vi "HexapodAcquireHardware.vi"(8 "error in (no error)":errorcluster, 11 "HexapodPI in":refnum<class "HexapodPI.lvclass">) -> (0 "error out":errorcluster, 1 "Status Cluster":T1, 2 "In Motion":bool, 3 "HexapodPI out":refnum<class "HexapodPI.lvclass">, 5 "Array":string[](array[string]))   [LabVIEW 2020, in "HexapodPI.lvclass"]
uses:
  HexapodPI.lvclass
  HexapodPI.lvclass/HexapodPI.ctl
  activeChannel.ctl
  OnOffTypeDef.ctl
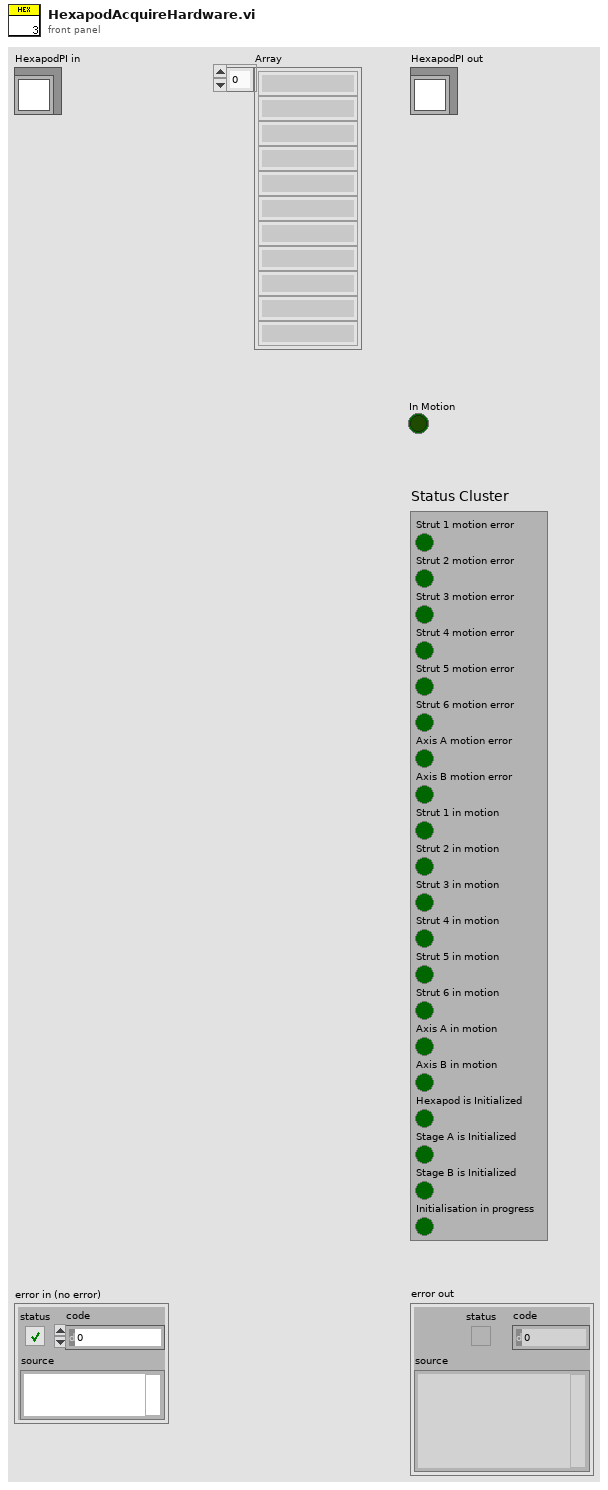
[diagram p1: front panel]
types:
  T1 = cluster{"Strut 1 motion error":bool, "Strut 2 motion error":bool, "Strut 3 motion error":bool, "Strut 4 motion error":bool, "Strut 5 motion error":bool, "Strut 6 motion error":bool, "Axis A motion error":bool, "Axis B motion error":bool, "Strut 1 in motion":bool, "Strut 2 in motion":bool, "Strut 3 in motion":bool, "Strut 4 in motion":bool, "Strut 5 in motion":bool, "Strut 6 in motion":bool, "Axis A in motion":bool, "Axis B in motion":bool, "Hexapod is Initialized":bool, "Stage A is Initialized":bool, "Stage B is Initialized":bool, "Initialisation in progress":bool}
  T2 = enum16{"Not referenced", "Homing", "Moving", "Ready"}
  T3 = typedef "OnOffTypeDef.ctl" = enum16{"off", "on"}
  T4 = cluster{"Zpos":T3, "Zneg":T3, "Xpos":T3, "Xneg":T3, "Ypos":T3, "Yneg":T3, "Wpos":T3, "Wneg":T3, "Vpos":T3, "Vneg":T3, "Upos":T3, "Uneg":T3}
  T5 = cluster{"connection ID":refnum<k5>, "VISA resource name":refnum<visa-resource-name>, "Selector":enum16{"TCPIP", "Serial"}}
  T6 = typedef "activeChannel.ctl" = enum16{"xpos", "ypos", "zpos", "uangle", "vangle", "wangle", "n/a", "off"}
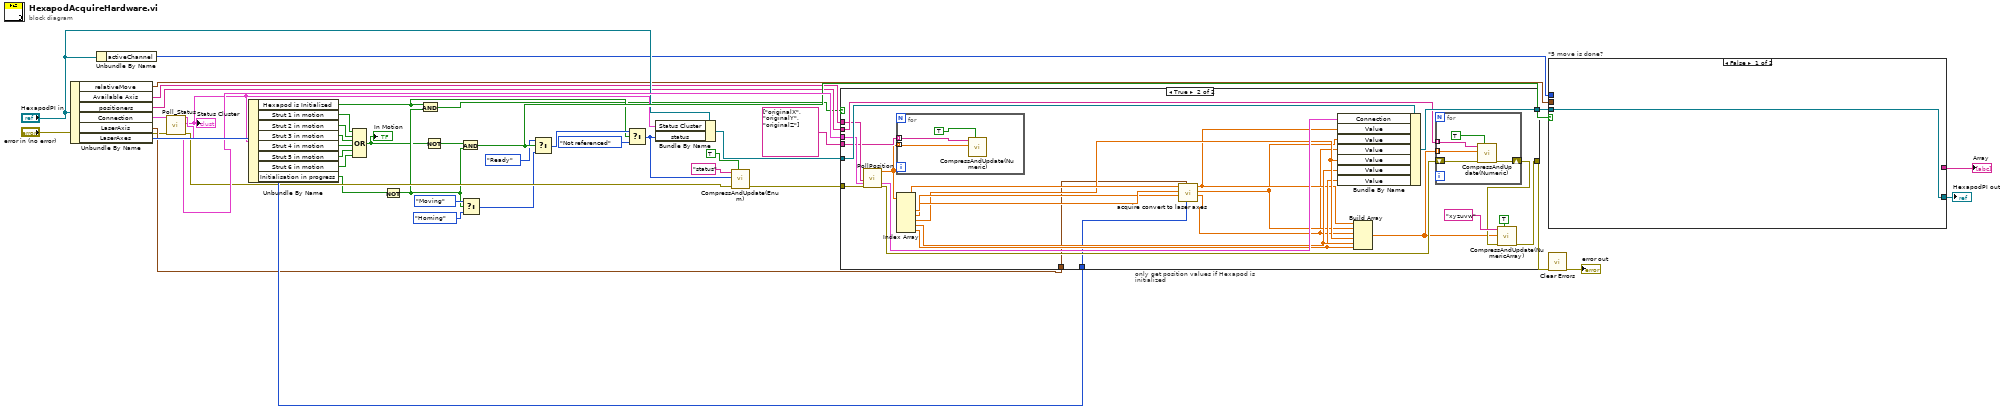
[diagram p0: block diagram]
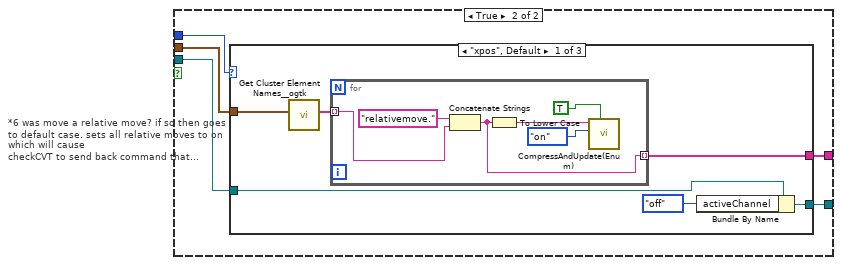
[diagram p2: hidden frame]
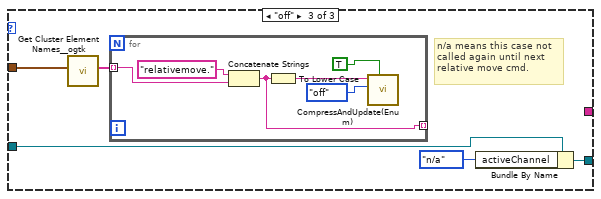
[diagram p4: hidden frame]
diagram:
  n1 = Unbundle By Name("HexapodPI in") -> ("relativeMove"=w33:T4, "Available Axis"=w28:string[], "positioners"=w27:string[], "Connection"=w2:T5, "LaserAxis"=w40:cluster{"u":dbl, "v":dbl, "w":dbl}, "LaserAxes"=w42:T3)
  n2 = Unbundle By Name("HexapodPI in") -> ("activeChannel"=w34:T6)
  n3 = call "Poll_Status.vi"("Connection"=w2, "error in"="error in (no error)") -> ("Connection out"=w41:T5, "Status Cluster"=w29:T1, "error out"=w22:errorcluster)  [unwired: 15 in]
  "Status Cluster" <- w29
  n4 = Unbundle By Name(w29) -> ("Hexapod is Initialized"=w19:bool, "Strut 1 in motion"=w10:bool, "Strut 2 in motion"=w5:bool, "Strut 3 in motion"=w6:bool, "Strut 4 in motion"=w7:bool, "Strut 5 in motion"=w8:bool, "Strut 6 in motion"=w9:bool, "Initialisation in progress"=w4:bool)
  n5 = Compound Arithmetic op=OR(w10, w5, w6, w7, w8, w9) -> (w14:bool)
  "In Motion" <- w14
  n6 = Not(x=w4) -> (.not. x?=w15:bool)
  n7 = And(x=w19, y=w15) -> (x .and. y?=w11:bool)
  n8 = Not(x=w14) -> (.not. x?=w32:bool)
  n9 = And(x=w32, y=w15) -> (x .and. y?=w38:bool)
  n10 = Select(t=T2."Moving" ("Settings.status"), s=w15, f=T2."Homing" ("Settings.status")) -> (s? t:f=w16:T2)
  n11 = Select(t=T2."Ready" ("Settings.status"), s=w38, f=w16) -> (s? t:f=w20:T2)
  n12 = Select(t=w20, s=w19, f=T2."Not referenced" ("Settings.status")) -> (s? t:f=w24:T2)
  n13 = Bundle By Name(cluster="HexapodPI in", "Status Cluster"=w29, "status"=w24) -> (w12:refnum<class "HexapodPI.lvclass">)
  n14 = call "CompressAndUpdate(Enum).vi"("force CVT update (false)"=TRUE, "error in"=w22, "enum variant"=w24, "command or variable name"="status") -> ("error out"=w23:errorcluster)  [unwired: 7 in]
  n15 = case "only get position values if Hexapod is initialized" shown="True" w11 {
    tunnel: [w43 w46] -> w30
    tunnel: [w44 w70] -> w36
    tunnel: w12 -> [w44 w69]
    tunnel: w23 -> [w43 w68]
    tunnel: w41 -> [_ w67]
    tunnel: w27 -> [_ w64]
    tunnel: w28 -> [_ w63]
    tunnel: string[] ["originalX", "originalY", "originalZ"] -> [_ w56]
    tunnel: w40 -> [_ w51]
    tunnel: w42 -> [_ w50]
    frame False {
    }
    frame True {
      n16 = call "PollPosition.vi"("Queried axes"=w63, "Connection"=w67, "error in"=w68) -> ("Position"=w55:dbl[], "Connection out"=w65:T5, "error out"=w66:errorcluster)  [unwired: 13 in, 1 out]
      n17 = for {
        tunnel: w55 -> [w72] mode=indexing
        tunnel: w56 -> [w71] mode=indexing
        n18 = call "CompressAndUpdate(Numeric).vi"("force CVT update (false)"=TRUE, "Numeric"=w72, "command or variable name"=w71) -> ()  [unwired: 8 in, 1 out]
      }
      n19 = Index Array(array=w55) -> (element #1=w62:dbl, element #2=w61:dbl, element #3=w60:dbl, element #4=w59:dbl, element #5=w58:dbl, element #6=w57:dbl)  [unwired: 6 in]
      n20 = call "acquire convert to laser axes.vi"("Settings.Trigger"=w50, "LaserAxis"=w51, "z in"=w60, "y in"=w61, "x in"=w62) -> ("z out"=w52:dbl, "y out"=w53:dbl, "x out"=w54:dbl)  [unwired: 4 in]
      n21 = Bundle By Name(cluster=w69, "Connection"=w65, "Value"=w54, "Value"=w53, "Value"=w52, "Value"=w59, "Value"=w58, "Value"=w57) -> (w70:refnum<class "HexapodPI.lvclass">)
      n22 = Build Array(w54, w53, w52, w59, w58, w57) -> (w45:dbl[])
      n23 = for {
        tunnel: w45 -> [w75] mode=indexing
        tunnel: w64 -> [w74] mode=indexing
        shift-right: [w78] -> w47
        shift-left: w66 -> [w76]
        n24 = call "CompressAndUpdate(Numeric).vi"("force CVT update (false)"=TRUE, "error in"=w76, "Numeric"=w75, "command or variable name"=w74) -> ("error out"=w78:errorcluster)  [unwired: 7 in]
      }
      n25 = call "CompressAndUpdate(NumericArray).vi"("force CVT update (false)"=TRUE, "error in"=w47, "Numeric Array"=w45, "command or variable name"="xyzuvw") -> ("error out"=w46:errorcluster)  [unwired: 7 in]
    }
  }
  n26 = case "*5 move is done?" shown="False" w38 {
    tunnel: w33 -> [_ w84]
    tunnel: w34 -> [_ w83]
    tunnel: w36 -> [w79 w82]
    tunnel: [w79 w81] -> w37
    tunnel: [_ w80] -> w1
    frame False {
    }
    frame True {
      n27 = case "*6 was move a relative move? if so then goes to default case. sets all relative moves to on which will cause\ncheckCVT to send back command that setrelative move was done. sets activechannel to off so next acquire will\nset all relative move enums to off." shown="\"xpos\", Default" w83 {
        tunnel: w84 -> [w90 _ w101]
        tunnel: w82 -> [w89 w97 w100]
        tunnel: [w88 w97 w98] -> w81
        tunnel: [w85 _ _] -> w80
        frame "xpos", Default {
          n28 = call "Get Cluster Element Names__ogtk.vi"("Cluster"=w90) -> ("Element Names"=w87:string[])  [unwired: 9 in, 1 out]
          n29 = for {
            tunnel: w87 -> [w96] mode=indexing
            tunnel: [w92] -> w85 mode=indexing
            n30 = Concatenate Strings("relativemove." ("string"), w96) -> (w92:string)
            n31 = To Lower Case(string=w92) -> (all lower case string=w91:string)
            n32 = call "CompressAndUpdate(Enum).vi"("force CVT update (false)"=TRUE, "enum variant"=OnOffTypeDef."on" ("Zpos"), "command or variable name"=w91) -> ()  [unwired: 8 in, 1 out]
          }
          n33 = Bundle By Name(cluster=w89, "activeChannel"=activeChannel."off") -> (w88:refnum<class "HexapodPI.lvclass">)
        }
        frame "n/a" {
        }
        frame "off" {
          # "n/a means this case not\ncalled again until next\nrelative move cmd."
          n34 = call "Get Cluster Element Names__ogtk.vi"("Cluster"=w101) -> ("Element Names"=w102:string[])  [unwired: 9 in, 1 out]
          n35 = for {
            tunnel: w102 -> [w108] mode=indexing
            tunnel: [w104] -> _ mode=indexing
            n36 = Concatenate Strings("relativemove." ("string"), w108) -> (w104:string)
            n37 = To Lower Case(string=w104) -> (all lower case string=w103:string)
            n38 = call "CompressAndUpdate(Enum).vi"("force CVT update (false)"=TRUE, "enum variant"=OnOffTypeDef."off" ("Zpos"), "command or variable name"=w103) -> ()  [unwired: 8 in, 1 out]
          }
          n39 = Bundle By Name(cluster=w100, "activeChannel"=activeChannel."n/a") -> (w98:refnum<class "HexapodPI.lvclass">)
        }
      }
    }
  }
  "HexapodPI out" <- w37
  "Array" <- w1
  n40 = call "Clear Errors.vi"("error in (no error)"=w30) -> ("error out"=→"error out":errorcluster)  [unwired: 5 in, 1 out]
